vi "Configure Joystick Button.vi"(6 "Command List":string[](array[string]), 7 "Event Type (1: pressed)":i32(ring)=1 items=["pressed"=1, "released before 1 second"=2, "held for 1 second"=3, "released after 1 second"=4], 8 "error in (no error)":errorcluster, 9 "Joystick Device Number":string, 10 "Key Index (1)":u8=1, 11 "VISA resource name":refnum<visa-resource-name>) -> (0 "error out":errorcluster, 3 "VISA resource name out":refnum<visa-resource-name>)   [LabVIEW 2015, in "Zaber A Series.lvlib"]
doc: "With VI you can configure the list of commands that a joystick will generate when one of its buttons is operated. \n\nYou must specify the device number of the joystick and the index of the key to configure. Different models of joystick may have different numbers of keys.\n\nYou should also select the specific key event that you want to fire the commands. Different lists of commands can be triggered by each of four key events: Initial press (1), release within a second (2), holding for a second (3), and releasing after more than a second (4).\n\nPass in an empty list of commands to clear the key event.\n\nThis VI expects the serial port to already have been configured."
uses:
  Zaber A Series.lvlib
  Private/All Commands.ctl
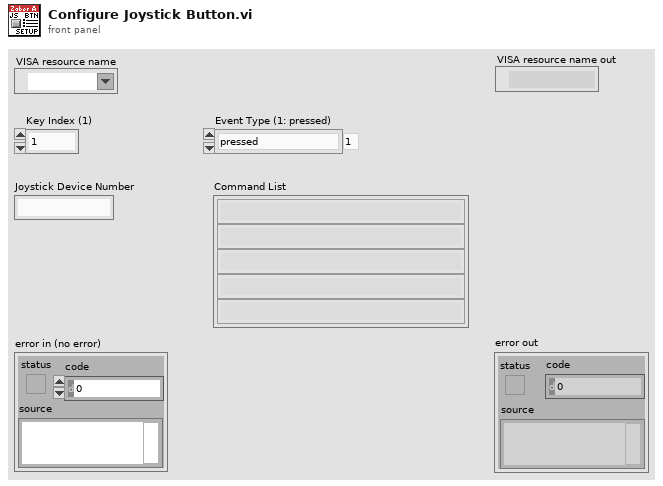
[diagram p1: front panel]
types:
  T1 = typedef "Zaber A Series.lvlib/All Commands.ctl" = string
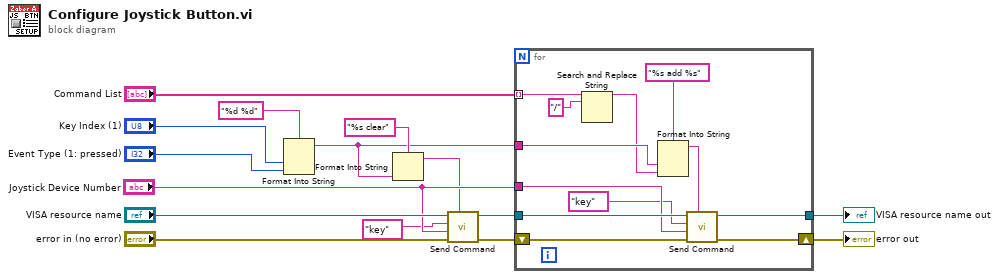
[diagram p0: block diagram]
diagram:
  n1 = Format Into String(format string="%d %d", "Key Index (1)", "Event Type (1: pressed)") -> (resulting string=w4:string)  [unwired: 2 in, 1 out]
  n2 = Format Into String(format string="%s clear", w4) -> (resulting string=w5:string)  [unwired: 2 in, 1 out]
  n3 = call "Send Command.vi"("Data"=w5, "error in (no error)"="error in (no error)", "Device and Axis"="Joystick Device Number", "Command"=T1 "key" ("Complete Command List"), "VISA resource name"="VISA resource name") -> ("error out"=w2:errorcluster, "VISA resource name out"=w3:refnum<visa-resource-name>)  [unwired: 1 in, 4 out]
  n4 = for {
    tunnel: "Command List" -> [w21] mode=indexing
    tunnel: "Joystick Device Number" -> [w25]
    shift-right: [w17] -> w11
    shift-left: w2 -> [w26]
    tunnel: w4 -> [w22]
    tunnel: w3 -> [w27]
    tunnel: [w18] -> w12
    n5 = Search and Replace String(input string=w21, search string="/") -> (result string=w20:string)  [unwired: 6 in, 3 out]
    n6 = Format Into String(format string="%s add %s", w22, w20) -> (resulting string=w23:string)  [unwired: 2 in, 1 out]
    n7 = call "Send Command.vi"("Data"=w23, "error in (no error)"=w26, "Device and Axis"=w25, "Command"=T1 "key" ("Complete Command List"), "VISA resource name"=w27) -> ("error out"=w17:errorcluster, "VISA resource name out"=w18:refnum<visa-resource-name>)  [unwired: 1 in, 4 out]
  }
  "VISA resource name out" <- w12
  "error out" <- w11
